vi "test.vi"() -> (10 "Array":dbl[](array[numeric]))   [LabVIEW 2010]
panel:
  in  "stop":bool
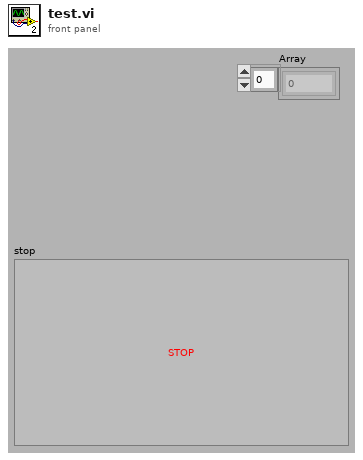
[diagram p1: front panel]
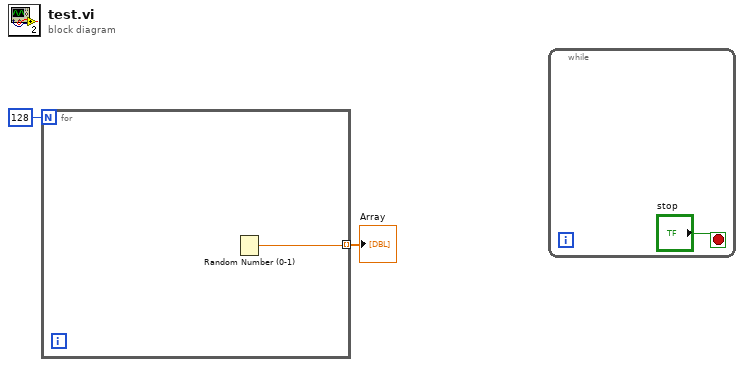
[diagram p0: block diagram]
diagram:
  n1 = for {
    N: 128 -> [_]
    tunnel: [w3] -> w1 mode=indexing
    n2 = Random Number (0-1)() -> (number: 0 to 1=w3:dbl)
  }
  "Array" <- w1
  n3 = while {
    stop <- "stop" stop-if-true
  }
